vi "Configure Module.vi"(8 "error in (no error)":errorcluster, 10 "IOV ref in":refnum<k21>, 11 "Module Template in":refnum<class "SD Module.lvclass">) -> (0 "error out":errorcluster, 2 "IOV ref out":refnum<k21>, 3 "Module Template out":refnum<class "SD Module.lvclass">)   [LabVIEW 2017, in "Modules.lvlib" / "SD Module.lvclass"]
uses:
  SD Module.lvclass
  C:/Users/nitest/Documents/ni-official/niveristand-scan-engine-module-libraries/Source/RSI Module/RSI Module.lvclass
  SD Module.lvclass/SD Module.ctl
  <resource>/objmgr/cRIO.rc
  RSI Module/RSI Module.lvclass
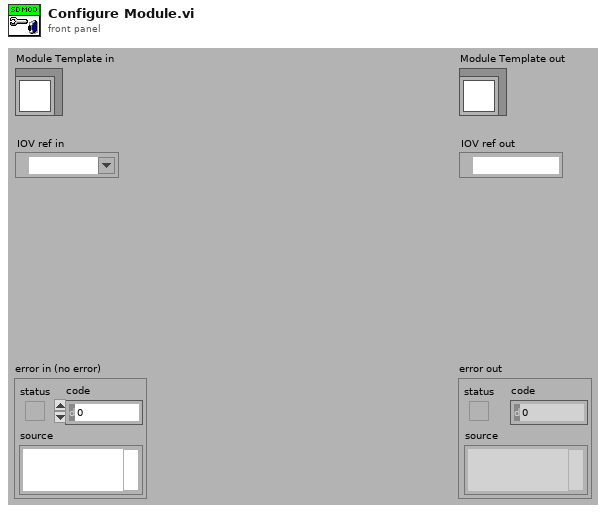
[diagram p1: front panel]
types:
  T1 = typedef "Modules.lvlib/SD Module.lvclass/Counter Channel.ctl" = cluster{"Measurement Mode":u32, "Count Edges":T2, "Period Measurement":T3, "Pulse Width Measurement":T4, "Frequency Measurement":T5}
  T2 = typedef "Modules.lvlib/SD Module.lvclass/Count Edges.ctl" = cluster{"Counter Event":u32, "Counter Source":u32, "Counter Direction":u32, "Terminal Count":u32, "Output Mode":u32, "Gate Mode":u32}
  T3 = typedef "Modules.lvlib/SD Module.lvclass/Period Measurement.ctl" = cluster{"Measurement Edge":u32}
  T4 = typedef "Modules.lvlib/SD Module.lvclass/Pulse Width Measurement.ctl" = cluster{"Measurement Type":u32}
  T5 = typedef "Modules.lvlib/SD Module.lvclass/Frequency Measurement.ctl" = cluster{"Measurement Edge":u32, "Measurement Timebase":u32}
  T6 = typedef "Modules.lvlib/SD Module.lvclass/CDO Channel.ctl" = cluster{"Counter driven enabled":bool}
  T7 = typedef "Modules.lvlib/SD Module.lvclass/PWM Channel.ctl" = cluster{"PWM frequency":u32}
  T8 = typedef "Modules.lvlib/SD Module.lvclass/Quadrature Channel.ctl" = cluster{"Timebase":u32, "Index Mode":u32}
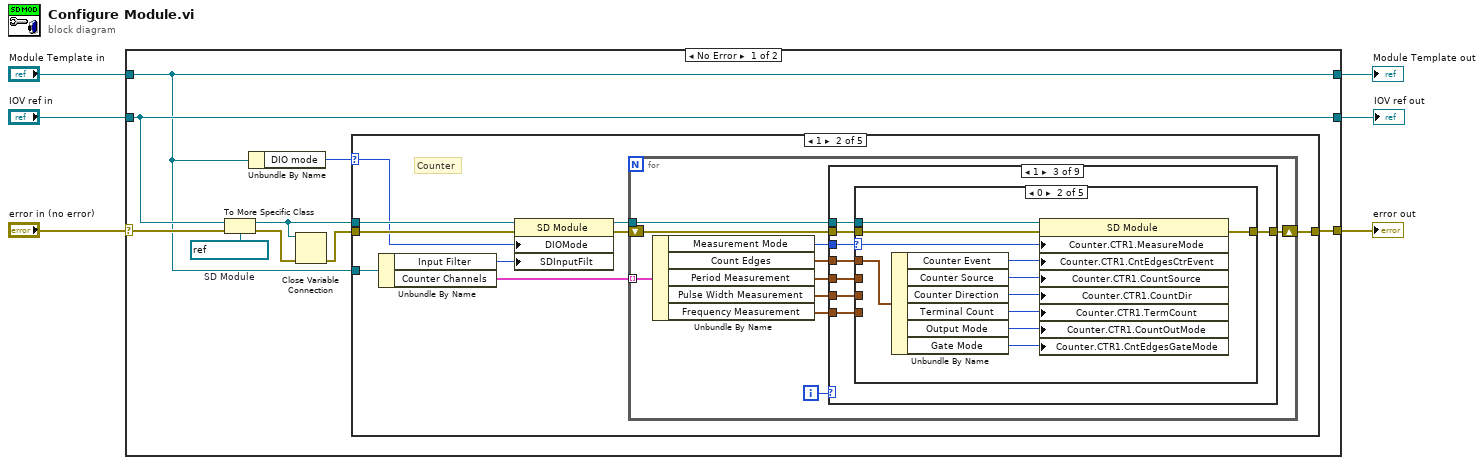
[diagram p0: block diagram]
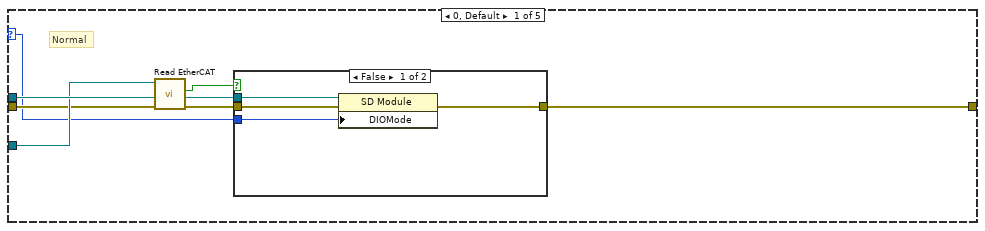
[diagram p2: hidden frame]
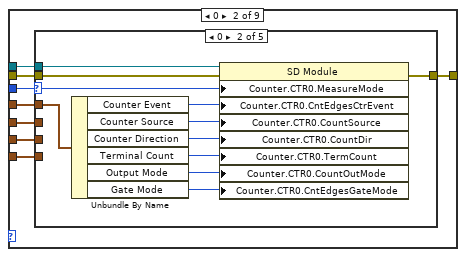
[diagram p5: hidden frame]
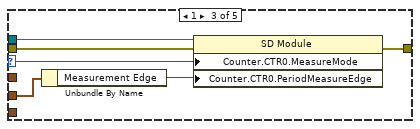
[diagram p7: hidden frame]
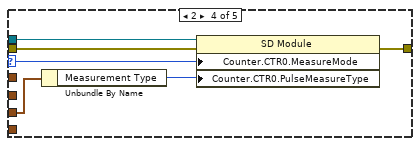
[diagram p8: hidden frame]
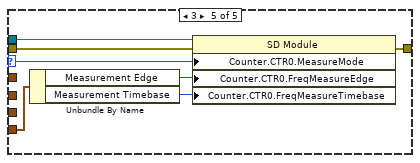
[diagram p9: hidden frame]
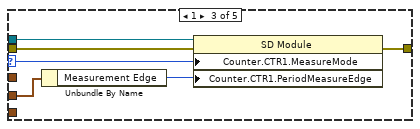
[diagram p11: hidden frame]
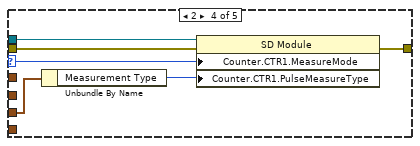
[diagram p12: hidden frame]
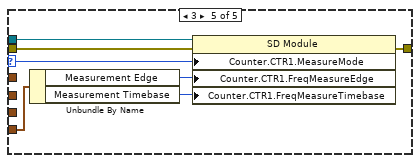
[diagram p13: hidden frame]
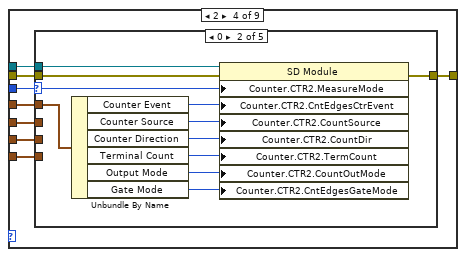
[diagram p14: hidden frame]
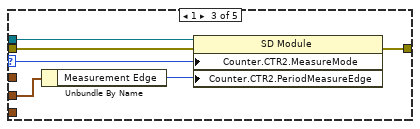
[diagram p16: hidden frame]
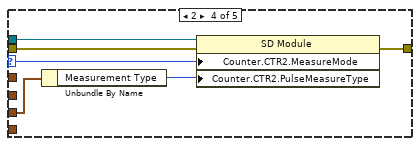
[diagram p17: hidden frame]
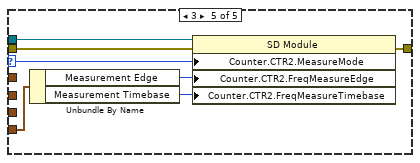
[diagram p18: hidden frame]
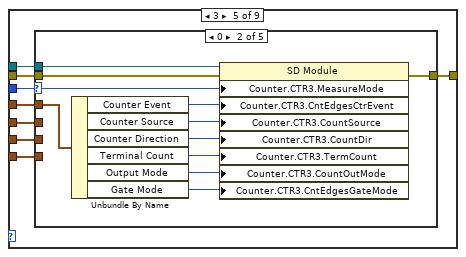
[diagram p19: hidden frame]
diagram:
  n1 = case shown="No Error" "error in (no error)" {
    selector: "error in (no error)" -> [w15 w484]
    tunnel: [w7 w484] -> w5
    tunnel: [w8 w483] -> w3
    tunnel: "Module Template in" -> [w8 w483]
    tunnel: "IOV ref in" -> [w13 w482]
    tunnel: [w13 w482] -> w1
    frame No Error {
      w14 = refnum<k21> refnum  # SD Module
      n2 = To More Specific Class(target class=w14, reference=w13, error in=w15) -> (specific class reference=w10:refnum<k21>, error out=w12:errorcluster)
      n3 = Unbundle By Name(w8) -> ("DIO mode"=w11:u32)
      n4 = Close Variable Connection(8:w12, 11:w10) -> (0:w9:errorcluster)
      n5 = case shown="1" w11 {
        selector: w11 -> [w16 w34 w366 w413 w461]
        tunnel: w10 -> [w22 w36 w368 w415 w463]
        tunnel: w9 -> [w18 w35 w367 w414 w462]
        tunnel: w8 -> [w20 w33 w365 w412 w460]
        tunnel: [w21 w28 w360 w408 w455] -> w7
        frame 0, Default {
          # "Normal"
          n6 = call "Read EtherCAT.vi"("error in (no error)"=w18, "RSI Module in"=w20) -> ("error out"=w17:errorcluster, "EtherCAT?"=w19:bool)  [unwired: 7 in, 1 out]
          n7 = case shown="False" w19 {
            tunnel: w22 -> [w26 _]
            tunnel: w17 -> [w25 w27]
            tunnel: [w24 w27] -> w21
            tunnel: w16 -> [w23 _]
            frame False {
              n8 = property class="SD Module"(reference=w26, error in=w25, "DIOMode"=w23) -> (error out=w24:errorcluster)  [unwired: 1 out]
            }
            frame True {
              # "Specialty Digital is not supported over\nEtherCAT, and explicitly configuring modules\nto use normal DIO mode will fail as a result."
            }
          }
        }
        frame 1 {
          # "Counter"
          n9 = Unbundle By Name(w33) -> ("Input Filter"=w32:u32, "Counter Channels"=w31:T1[])
          n10 = property class="SD Module"(reference=w36, error in=w35, "DIOMode"=w34, "SDInputFilt"=w32) -> (reference out=w30:refnum<k21>, error out=w29:errorcluster)
          n11 = for {
            tunnel: w31 -> [w42] mode=indexing
            tunnel: w30 -> [w45]
            shift-right: [w43] -> w28
            shift-left: w29 -> [w44]
            i -> [w46]
            n12 = Unbundle By Name(w42) -> ("Measurement Mode"=w41:u32, "Count Edges"=w40:T2, "Period Measurement"=w39:T3, "Pulse Width Measurement"=w38:T4, "Frequency Measurement"=w37:T5)
            n13 = case shown="1" w46 {
              tunnel: w45 -> [_ w50 w89 w128 w167 w206 w245 w284 w323]
              tunnel: w44 -> [w47 w49 w88 w127 w166 w205 w244 w283 w322]
              tunnel: [w47 w48 w87 w126 w165 w204 w243 w282 w321] -> w43
              tunnel: w41 -> [_ w55 w94 w133 w172 w211 w250 w289 w328]
              tunnel: w40 -> [_ w54 w93 w132 w171 w210 w249 w288 w327]
              tunnel: w39 -> [_ w53 w92 w131 w170 w209 w248 w287 w326]
              tunnel: w38 -> [_ w52 w91 w130 w169 w208 w247 w286 w325]
              tunnel: w37 -> [_ w51 w90 w129 w168 w207 w246 w285 w324]
              frame Default {
              }
              frame 0 {
                n14 = case shown="0" w55 {
                  selector: w55 -> [_ w64 w71 w77 w84]
                  tunnel: w54 -> [_ w67 _ _ _]
                  tunnel: w53 -> [_ _ w68 _ _]
                  tunnel: w52 -> [_ _ _ w74 _]
                  tunnel: w51 -> [_ _ _ _ w81]
                  tunnel: w50 -> [_ w66 w73 w79 w86]
                  tunnel: w49 -> [w56 w65 w72 w78 w85]
                  tunnel: [w56 w57 w69 w75 w82] -> w48
                  frame Default {
                  }
                  frame 0 {
                    n15 = Unbundle By Name(w67) -> ("Counter Event"=w63:u32, "Counter Source"=w62:u32, "Counter Direction"=w61:u32, "Terminal Count"=w60:u32, "Output Mode"=w59:u32, "Gate Mode"=w58:u32)
                    n16 = property class="SD Module"(reference=w66, error in=w65, "Counter.CTR0.MeasureMode"=w64, "Counter.CTR0.CntEdgesCtrEvent"=w63, "Counter.CTR0.CountSource"=w62, "Counter.CTR0.CountDir"=w61, "Counter.CTR0.TermCount"=w60, "Counter.CTR0.CountOutMode"=w59, "Counter.CTR0.CntEdgesGateMode"=w58) -> (error out=w57:errorcluster)  [unwired: 1 out]
                  }
                  frame 1 {
                    n17 = Unbundle By Name(w68) -> ("Measurement Edge"=w70:u32)
                    n18 = property class="SD Module"(reference=w73, error in=w72, "Counter.CTR0.MeasureMode"=w71, "Counter.CTR0.PeriodMeasureEdge"=w70) -> (error out=w69:errorcluster)  [unwired: 1 out]
                  }
                  frame 2 {
                    n19 = Unbundle By Name(w74) -> ("Measurement Type"=w76:u32)
                    n20 = property class="SD Module"(reference=w79, error in=w78, "Counter.CTR0.MeasureMode"=w77, "Counter.CTR0.PulseMeasureType"=w76) -> (error out=w75:errorcluster)  [unwired: 1 out]
                  }
                  frame 3 {
                    n21 = Unbundle By Name(w81) -> ("Measurement Edge"=w83:u32, "Measurement Timebase"=w80:u32)
                    n22 = property class="SD Module"(reference=w86, error in=w85, "Counter.CTR0.MeasureMode"=w84, "Counter.CTR0.FreqMeasureEdge"=w83, "Counter.CTR0.FreqMeasureTimebase"=w80) -> (error out=w82:errorcluster)  [unwired: 1 out]
                  }
                }
              }
              frame 1 {
                n23 = case shown="0" w94 {
                  selector: w94 -> [_ w103 w110 w116 w123]
                  tunnel: w93 -> [_ w106 _ _ _]
                  tunnel: w92 -> [_ _ w107 _ _]
                  tunnel: w91 -> [_ _ _ w113 _]
                  tunnel: w90 -> [_ _ _ _ w120]
                  tunnel: w89 -> [_ w105 w112 w118 w125]
                  tunnel: w88 -> [w95 w104 w111 w117 w124]
                  tunnel: [w95 w96 w108 w114 w121] -> w87
                  frame Default {
                  }
                  frame 0 {
                    n24 = Unbundle By Name(w106) -> ("Counter Event"=w102:u32, "Counter Source"=w101:u32, "Counter Direction"=w100:u32, "Terminal Count"=w99:u32, "Output Mode"=w98:u32, "Gate Mode"=w97:u32)
                    n25 = property class="SD Module"(reference=w105, error in=w104, "Counter.CTR1.MeasureMode"=w103, "Counter.CTR1.CntEdgesCtrEvent"=w102, "Counter.CTR1.CountSource"=w101, "Counter.CTR1.CountDir"=w100, "Counter.CTR1.TermCount"=w99, "Counter.CTR1.CountOutMode"=w98, "Counter.CTR1.CntEdgesGateMode"=w97) -> (error out=w96:errorcluster)  [unwired: 1 out]
                  }
                  frame 1 {
                    n26 = Unbundle By Name(w107) -> ("Measurement Edge"=w109:u32)
                    n27 = property class="SD Module"(reference=w112, error in=w111, "Counter.CTR1.MeasureMode"=w110, "Counter.CTR1.PeriodMeasureEdge"=w109) -> (error out=w108:errorcluster)  [unwired: 1 out]
                  }
                  frame 2 {
                    n28 = Unbundle By Name(w113) -> ("Measurement Type"=w115:u32)
                    n29 = property class="SD Module"(reference=w118, error in=w117, "Counter.CTR1.MeasureMode"=w116, "Counter.CTR1.PulseMeasureType"=w115) -> (error out=w114:errorcluster)  [unwired: 1 out]
                  }
                  frame 3 {
                    n30 = Unbundle By Name(w120) -> ("Measurement Edge"=w122:u32, "Measurement Timebase"=w119:u32)
                    n31 = property class="SD Module"(reference=w125, error in=w124, "Counter.CTR1.MeasureMode"=w123, "Counter.CTR1.FreqMeasureEdge"=w122, "Counter.CTR1.FreqMeasureTimebase"=w119) -> (error out=w121:errorcluster)  [unwired: 1 out]
                  }
                }
              }
              frame 2 {
                n32 = case shown="0" w133 {
                  selector: w133 -> [_ w142 w149 w155 w162]
                  tunnel: w132 -> [_ w145 _ _ _]
                  tunnel: w131 -> [_ _ w146 _ _]
                  tunnel: w130 -> [_ _ _ w152 _]
                  tunnel: w129 -> [_ _ _ _ w159]
                  tunnel: w128 -> [_ w144 w151 w157 w164]
                  tunnel: w127 -> [w134 w143 w150 w156 w163]
                  tunnel: [w134 w135 w147 w153 w160] -> w126
                  frame Default {
                  }
                  frame 0 {
                    n33 = Unbundle By Name(w145) -> ("Counter Event"=w141:u32, "Counter Source"=w140:u32, "Counter Direction"=w139:u32, "Terminal Count"=w138:u32, "Output Mode"=w137:u32, "Gate Mode"=w136:u32)
                    n34 = property class="SD Module"(reference=w144, error in=w143, "Counter.CTR2.MeasureMode"=w142, "Counter.CTR2.CntEdgesCtrEvent"=w141, "Counter.CTR2.CountSource"=w140, "Counter.CTR2.CountDir"=w139, "Counter.CTR2.TermCount"=w138, "Counter.CTR2.CountOutMode"=w137, "Counter.CTR2.CntEdgesGateMode"=w136) -> (error out=w135:errorcluster)  [unwired: 1 out]
                  }
                  frame 1 {
                    n35 = Unbundle By Name(w146) -> ("Measurement Edge"=w148:u32)
                    n36 = property class="SD Module"(reference=w151, error in=w150, "Counter.CTR2.MeasureMode"=w149, "Counter.CTR2.PeriodMeasureEdge"=w148) -> (error out=w147:errorcluster)  [unwired: 1 out]
                  }
                  frame 2 {
                    n37 = Unbundle By Name(w152) -> ("Measurement Type"=w154:u32)
                    n38 = property class="SD Module"(reference=w157, error in=w156, "Counter.CTR2.MeasureMode"=w155, "Counter.CTR2.PulseMeasureType"=w154) -> (error out=w153:errorcluster)  [unwired: 1 out]
                  }
                  frame 3 {
                    n39 = Unbundle By Name(w159) -> ("Measurement Edge"=w161:u32, "Measurement Timebase"=w158:u32)
                    n40 = property class="SD Module"(reference=w164, error in=w163, "Counter.CTR2.MeasureMode"=w162, "Counter.CTR2.FreqMeasureEdge"=w161, "Counter.CTR2.FreqMeasureTimebase"=w158) -> (error out=w160:errorcluster)  [unwired: 1 out]
                  }
                }
              }
              frame 3 {
                n41 = case shown="0" w172 {
                  selector: w172 -> [_ w181 w188 w194 w201]
                  tunnel: w171 -> [_ w184 _ _ _]
                  tunnel: w170 -> [_ _ w185 _ _]
                  tunnel: w169 -> [_ _ _ w191 _]
                  tunnel: w168 -> [_ _ _ _ w198]
                  tunnel: w167 -> [_ w183 w190 w196 w203]
                  tunnel: w166 -> [w173 w182 w189 w195 w202]
                  tunnel: [w173 w174 w186 w192 w199] -> w165
                  frame Default {
                  }
                  frame 0 {
                    n42 = Unbundle By Name(w184) -> ("Counter Event"=w180:u32, "Counter Source"=w179:u32, "Counter Direction"=w178:u32, "Terminal Count"=w177:u32, "Output Mode"=w176:u32, "Gate Mode"=w175:u32)
                    n43 = property class="SD Module"(reference=w183, error in=w182, "Counter.CTR3.MeasureMode"=w181, "Counter.CTR3.CntEdgesCtrEvent"=w180, "Counter.CTR3.CountSource"=w179, "Counter.CTR3.CountDir"=w178, "Counter.CTR3.TermCount"=w177, "Counter.CTR3.CountOutMode"=w176, "Counter.CTR3.CntEdgesGateMode"=w175) -> (error out=w174:errorcluster)  [unwired: 1 out]
                  }
                  frame 1 {
                    n44 = Unbundle By Name(w185) -> ("Measurement Edge"=w187:u32)
                    n45 = property class="SD Module"(reference=w190, error in=w189, "Counter.CTR3.MeasureMode"=w188, "Counter.CTR3.PeriodMeasureEdge"=w187) -> (error out=w186:errorcluster)  [unwired: 1 out]
                  }
                  frame 2 {
                    n46 = Unbundle By Name(w191) -> ("Measurement Type"=w193:u32)
                    n47 = property class="SD Module"(reference=w196, error in=w195, "Counter.CTR3.MeasureMode"=w194, "Counter.CTR3.PulseMeasureType"=w193) -> (error out=w192:errorcluster)  [unwired: 1 out]
                  }
                  frame 3 {
                    n48 = Unbundle By Name(w198) -> ("Measurement Edge"=w200:u32, "Measurement Timebase"=w197:u32)
                    n49 = property class="SD Module"(reference=w203, error in=w202, "Counter.CTR3.MeasureMode"=w201, "Counter.CTR3.FreqMeasureEdge"=w200, "Counter.CTR3.FreqMeasureTimebase"=w197) -> (error out=w199:errorcluster)  [unwired: 1 out]
                  }
                }
              }
              frame 4 {
                n50 = case shown="0" w211 {
                  selector: w211 -> [_ w220 w227 w233 w240]
                  tunnel: w210 -> [_ w223 _ _ _]
                  tunnel: w209 -> [_ _ w224 _ _]
                  tunnel: w208 -> [_ _ _ w230 _]
                  tunnel: w207 -> [_ _ _ _ w237]
                  tunnel: w206 -> [_ w222 w229 w235 w242]
                  tunnel: w205 -> [w212 w221 w228 w234 w241]
                  tunnel: [w212 w213 w225 w231 w238] -> w204
                  frame Default {
                  }
                  frame 0 {
                    n51 = Unbundle By Name(w223) -> ("Counter Event"=w219:u32, "Counter Source"=w218:u32, "Counter Direction"=w217:u32, "Terminal Count"=w216:u32, "Output Mode"=w215:u32, "Gate Mode"=w214:u32)
                    n52 = property class="SD Module"(reference=w222, error in=w221, "Counter.CTR4.MeasureMode"=w220, "Counter.CTR4.CntEdgesCtrEvent"=w219, "Counter.CTR4.CountSource"=w218, "Counter.CTR4.CountDir"=w217, "Counter.CTR4.TermCount"=w216, "Counter.CTR4.CountOutMode"=w215, "Counter.CTR4.CntEdgesGateMode"=w214) -> (error out=w213:errorcluster)  [unwired: 1 out]
                  }
                  frame 1 {
                    n53 = Unbundle By Name(w224) -> ("Measurement Edge"=w226:u32)
                    n54 = property class="SD Module"(reference=w229, error in=w228, "Counter.CTR4.MeasureMode"=w227, "Counter.CTR4.PeriodMeasureEdge"=w226) -> (error out=w225:errorcluster)  [unwired: 1 out]
                  }
                  frame 2 {
                    n55 = Unbundle By Name(w230) -> ("Measurement Type"=w232:u32)
                    n56 = property class="SD Module"(reference=w235, error in=w234, "Counter.CTR4.MeasureMode"=w233, "Counter.CTR4.PulseMeasureType"=w232) -> (error out=w231:errorcluster)  [unwired: 1 out]
                  }
                  frame 3 {
                    n57 = Unbundle By Name(w237) -> ("Measurement Edge"=w239:u32, "Measurement Timebase"=w236:u32)
                    n58 = property class="SD Module"(reference=w242, error in=w241, "Counter.CTR4.MeasureMode"=w240, "Counter.CTR4.FreqMeasureEdge"=w239, "Counter.CTR4.FreqMeasureTimebase"=w236) -> (error out=w238:errorcluster)  [unwired: 1 out]
                  }
                }
              }
              frame 5 {
                n59 = case shown="0" w250 {
                  selector: w250 -> [_ w259 w266 w272 w279]
                  tunnel: w249 -> [_ w262 _ _ _]
                  tunnel: w248 -> [_ _ w263 _ _]
                  tunnel: w247 -> [_ _ _ w269 _]
                  tunnel: w246 -> [_ _ _ _ w276]
                  tunnel: w245 -> [_ w261 w268 w274 w281]
                  tunnel: w244 -> [w251 w260 w267 w273 w280]
                  tunnel: [w251 w252 w264 w270 w277] -> w243
                  frame Default {
                  }
                  frame 0 {
                    n60 = Unbundle By Name(w262) -> ("Counter Event"=w258:u32, "Counter Source"=w257:u32, "Counter Direction"=w256:u32, "Terminal Count"=w255:u32, "Output Mode"=w254:u32, "Gate Mode"=w253:u32)
                    n61 = property class="SD Module"(reference=w261, error in=w260, "Counter.CTR5.MeasureMode"=w259, "Counter.CTR5.CntEdgesCtrEvent"=w258, "Counter.CTR5.CountSource"=w257, "Counter.CTR5.CountDir"=w256, "Counter.CTR5.TermCount"=w255, "Counter.CTR5.CountOutMode"=w254, "Counter.CTR5.CntEdgesGateMode"=w253) -> (error out=w252:errorcluster)  [unwired: 1 out]
                  }
                  frame 1 {
                    n62 = Unbundle By Name(w263) -> ("Measurement Edge"=w265:u32)
                    n63 = property class="SD Module"(reference=w268, error in=w267, "Counter.CTR5.MeasureMode"=w266, "Counter.CTR5.PeriodMeasureEdge"=w265) -> (error out=w264:errorcluster)  [unwired: 1 out]
                  }
                  frame 2 {
                    n64 = Unbundle By Name(w269) -> ("Measurement Type"=w271:u32)
                    n65 = property class="SD Module"(reference=w274, error in=w273, "Counter.CTR5.MeasureMode"=w272, "Counter.CTR5.PulseMeasureType"=w271) -> (error out=w270:errorcluster)  [unwired: 1 out]
                  }
                  frame 3 {
                    n66 = Unbundle By Name(w276) -> ("Measurement Edge"=w278:u32, "Measurement Timebase"=w275:u32)
                    n67 = property class="SD Module"(reference=w281, error in=w280, "Counter.CTR5.MeasureMode"=w279, "Counter.CTR5.FreqMeasureEdge"=w278, "Counter.CTR5.FreqMeasureTimebase"=w275) -> (error out=w277:errorcluster)  [unwired: 1 out]
                  }
                }
              }
              frame 6 {
                n68 = case shown="0" w289 {
                  selector: w289 -> [_ w298 w305 w311 w318]
                  tunnel: w288 -> [_ w301 _ _ _]
                  tunnel: w287 -> [_ _ w302 _ _]
                  tunnel: w286 -> [_ _ _ w308 _]
                  tunnel: w285 -> [_ _ _ _ w315]
                  tunnel: w284 -> [_ w300 w307 w313 w320]
                  tunnel: w283 -> [w290 w299 w306 w312 w319]
                  tunnel: [w290 w291 w303 w309 w316] -> w282
                  frame Default {
                  }
                  frame 0 {
                    n69 = Unbundle By Name(w301) -> ("Counter Event"=w297:u32, "Counter Source"=w296:u32, "Counter Direction"=w295:u32, "Terminal Count"=w294:u32, "Output Mode"=w293:u32, "Gate Mode"=w292:u32)
                    n70 = property class="SD Module"(reference=w300, error in=w299, "Counter.CTR6.MeasureMode"=w298, "Counter.CTR6.CntEdgesCtrEvent"=w297, "Counter.CTR6.CountSource"=w296, "Counter.CTR6.CountDir"=w295, "Counter.CTR6.TermCount"=w294, "Counter.CTR6.CountOutMode"=w293, "Counter.CTR6.CntEdgesGateMode"=w292) -> (error out=w291:errorcluster)  [unwired: 1 out]
                  }
                  frame 1 {
                    n71 = Unbundle By Name(w302) -> ("Measurement Edge"=w304:u32)
                    n72 = property class="SD Module"(reference=w307, error in=w306, "Counter.CTR6.MeasureMode"=w305, "Counter.CTR6.PeriodMeasureEdge"=w304) -> (error out=w303:errorcluster)  [unwired: 1 out]
                  }
                  frame 2 {
                    n73 = Unbundle By Name(w308) -> ("Measurement Type"=w310:u32)
                    n74 = property class="SD Module"(reference=w313, error in=w312, "Counter.CTR6.MeasureMode"=w311, "Counter.CTR6.PulseMeasureType"=w310) -> (error out=w309:errorcluster)  [unwired: 1 out]
                  }
                  frame 3 {
                    n75 = Unbundle By Name(w315) -> ("Measurement Edge"=w317:u32, "Measurement Timebase"=w314:u32)
                    n76 = property class="SD Module"(reference=w320, error in=w319, "Counter.CTR6.MeasureMode"=w318, "Counter.CTR6.FreqMeasureEdge"=w317, "Counter.CTR6.FreqMeasureTimebase"=w314) -> (error out=w316:errorcluster)  [unwired: 1 out]
                  }
                }
              }
              frame 7 {
                n77 = case shown="0" w328 {
                  selector: w328 -> [_ w337 w344 w350 w357]
                  tunnel: w327 -> [_ w340 _ _ _]
                  tunnel: w326 -> [_ _ w341 _ _]
                  tunnel: w325 -> [_ _ _ w347 _]
                  tunnel: w324 -> [_ _ _ _ w354]
                  tunnel: w323 -> [_ w339 w346 w352 w359]
                  tunnel: w322 -> [w329 w338 w345 w351 w358]
                  tunnel: [w329 w330 w342 w348 w355] -> w321
                  frame Default {
                  }
                  frame 0 {
                    n78 = Unbundle By Name(w340) -> ("Counter Event"=w336:u32, "Counter Source"=w335:u32, "Counter Direction"=w334:u32, "Terminal Count"=w333:u32, "Output Mode"=w332:u32, "Gate Mode"=w331:u32)
                    n79 = property class="SD Module"(reference=w339, error in=w338, "Counter.CTR7.MeasureMode"=w337, "Counter.CTR7.CntEdgesCtrEvent"=w336, "Counter.CTR7.CountSource"=w335, "Counter.CTR7.CountDir"=w334, "Counter.CTR7.TermCount"=w333, "Counter.CTR7.CountOutMode"=w332, "Counter.CTR7.CntEdgesGateMode"=w331) -> (error out=w330:errorcluster)  [unwired: 1 out]
                  }
                  frame 1 {
                    n80 = Unbundle By Name(w341) -> ("Measurement Edge"=w343:u32)
                    n81 = property class="SD Module"(reference=w346, error in=w345, "Counter.CTR7.MeasureMode"=w344, "Counter.CTR7.PeriodMeasureEdge"=w343) -> (error out=w342:errorcluster)  [unwired: 1 out]
                  }
                  frame 2 {
                    n82 = Unbundle By Name(w347) -> ("Measurement Type"=w349:u32)
                    n83 = property class="SD Module"(reference=w352, error in=w351, "Counter.CTR7.MeasureMode"=w350, "Counter.CTR7.PulseMeasureType"=w349) -> (error out=w348:errorcluster)  [unwired: 1 out]
                  }
                  frame 3 {
                    n84 = Unbundle By Name(w354) -> ("Measurement Edge"=w356:u32, "Measurement Timebase"=w353:u32)
                    n85 = property class="SD Module"(reference=w359, error in=w358, "Counter.CTR7.MeasureMode"=w357, "Counter.CTR7.FreqMeasureEdge"=w356, "Counter.CTR7.FreqMeasureTimebase"=w353) -> (error out=w355:errorcluster)  [unwired: 1 out]
                  }
                }
              }
            }
          }
        }
        frame 2 {
          # "Counter-Driven Output"
          n86 = Unbundle By Name(w365) -> ("Drive From Slot"=w362:u32, "CDO Channels"=w361:T6[])
          n87 = property class="SD Module"(reference=w368, error in=w367, "DIOMode"=w366, "CDO.CountSlvMastSlot"=w362) -> (reference out=w364:refnum<k21>, error out=w363:errorcluster)
          n88 = for {
            tunnel: w364 -> [w373]
            shift-right: [w371] -> w360
            shift-left: w363 -> [w372]
            tunnel: w361 -> [w369] mode=indexing
            i -> [w374]
            n89 = Unbundle By Name(w369) -> ("Counter driven enabled"=w370:bool)
            n90 = case shown="0" w374 {
              tunnel: w373 -> [_ w379 w383 w387 w391 w395 w399 w403 w407]
              tunnel: w372 -> [w375 w378 w382 w386 w390 w394 w398 w402 w406]
              tunnel: [w375 w377 w381 w385 w389 w393 w397 w401 w405] -> w371
              tunnel: w370 -> [_ w376 w380 w384 w388 w392 w396 w400 w404]
              frame Default {
              }
              frame 0 {
                n91 = property class="SD Module"(reference=w379, error in=w378, "CDO.CTR0.CtrDrivenEnabled"=w376) -> (error out=w377:errorcluster)  [unwired: 1 out]
              }
              frame 1 {
                n92 = property class="SD Module"(reference=w383, error in=w382, "CDO.CTR1.CtrDrivenEnabled"=w380) -> (error out=w381:errorcluster)  [unwired: 1 out]
              }
              frame 2 {
                n93 = property class="SD Module"(reference=w387, error in=w386, "CDO.CTR2.CtrDrivenEnabled"=w384) -> (error out=w385:errorcluster)  [unwired: 1 out]
              }
              frame 3 {
                n94 = property class="SD Module"(reference=w391, error in=w390, "CDO.CTR3.CtrDrivenEnabled"=w388) -> (error out=w389:errorcluster)  [unwired: 1 out]
              }
              frame 4 {
                n95 = property class="SD Module"(reference=w395, error in=w394, "CDO.CTR4.CtrDrivenEnabled"=w392) -> (error out=w393:errorcluster)  [unwired: 1 out]
              }
              frame 5 {
                n96 = property class="SD Module"(reference=w399, error in=w398, "CDO.CTR5.CtrDrivenEnabled"=w396) -> (error out=w397:errorcluster)  [unwired: 1 out]
              }
              frame 6 {
                n97 = property class="SD Module"(reference=w403, error in=w402, "CDO.CTR6.CtrDrivenEnabled"=w400) -> (error out=w401:errorcluster)  [unwired: 1 out]
              }
              frame 7 {
                n98 = property class="SD Module"(reference=w407, error in=w406, "CDO.CTR7.CtrDrivenEnabled"=w404) -> (error out=w405:errorcluster)  [unwired: 1 out]
              }
            }
          }
        }
        frame 3 {
          # "Pulse-Width Modulation"
          n99 = Unbundle By Name(w412) -> ("PWM Channels"=w409:T7[])
          n100 = property class="SD Module"(reference=w415, error in=w414, "DIOMode"=w413) -> (reference out=w411:refnum<k21>, error out=w410:errorcluster)
          n101 = for {
            tunnel: w411 -> [w420]
            shift-right: [w418] -> w408
            shift-left: w410 -> [w419]
            tunnel: w409 -> [w416] mode=indexing
            i -> [w421]
            n102 = Unbundle By Name(w416) -> ("PWM frequency"=w417:u32)
            n103 = case shown="0" w421 {
              tunnel: w420 -> [_ w426 w430 w434 w438 w442 w446 w450 w454]
              tunnel: w419 -> [w422 w425 w429 w433 w437 w441 w445 w449 w453]
              tunnel: [w422 w424 w428 w432 w436 w440 w444 w448 w452] -> w418
              tunnel: w417 -> [_ w423 w427 w431 w435 w439 w443 w447 w451]
              frame Default {
              }
              frame 0 {
                n104 = property class="SD Module"(reference=w426, error in=w425, "PWM.PWM0.PWMFrequency"=w423) -> (error out=w424:errorcluster)  [unwired: 1 out]
              }
              frame 1 {
                n105 = property class="SD Module"(reference=w430, error in=w429, "PWM.PWM1.PWMFrequency"=w427) -> (error out=w428:errorcluster)  [unwired: 1 out]
              }
              frame 2 {
                n106 = property class="SD Module"(reference=w434, error in=w433, "PWM.PWM2.PWMFrequency"=w431) -> (error out=w432:errorcluster)  [unwired: 1 out]
              }
              frame 3 {
                n107 = property class="SD Module"(reference=w438, error in=w437, "PWM.PWM3.PWMFrequency"=w435) -> (error out=w436:errorcluster)  [unwired: 1 out]
              }
              frame 4 {
                n108 = property class="SD Module"(reference=w442, error in=w441, "PWM.PWM4.PWMFrequency"=w439) -> (error out=w440:errorcluster)  [unwired: 1 out]
              }
              frame 5 {
                n109 = property class="SD Module"(reference=w446, error in=w445, "PWM.PWM5.PWMFrequency"=w443) -> (error out=w444:errorcluster)  [unwired: 1 out]
              }
              frame 6 {
                n110 = property class="SD Module"(reference=w450, error in=w449, "PWM.PWM6.PWMFrequency"=w447) -> (error out=w448:errorcluster)  [unwired: 1 out]
              }
              frame 7 {
                n111 = property class="SD Module"(reference=w454, error in=w453, "PWM.PWM7.PWMFrequency"=w451) -> (error out=w452:errorcluster)  [unwired: 1 out]
              }
            }
          }
        }
        frame 4 {
          # "Quadrature"
          n112 = Unbundle By Name(w460) -> ("Input Filter"=w459:u32, "Quadrature Channels"=w458:T8[])
          n113 = property class="SD Module"(reference=w463, error in=w462, "DIOMode"=w461, "SDInputFilt"=w459) -> (reference out=w457:refnum<k21>, error out=w456:errorcluster)
          n114 = for {
            tunnel: w458 -> [w466] mode=indexing
            tunnel: w457 -> [w469]
            shift-right: [w467] -> w455
            shift-left: w456 -> [w468]
            i -> [w470]
            n115 = Unbundle By Name(w466) -> ("Timebase"=w465:u32, "Index Mode"=w464:u32)
            n116 = case shown="0" w470 {
              tunnel: w469 -> [_ w476 w481]
              tunnel: w468 -> [w471 w475 w480]
              tunnel: [w471 w474 w479] -> w467
              tunnel: w465 -> [_ w473 w478]
              tunnel: w464 -> [_ w472 w477]
              frame Default {
              }
              frame 0 {
                n117 = property class="SD Module"(reference=w476, error in=w475, "Quad.Quadrature0.QuadTimebase"=w473, "Quad.Quadrature0.QuadIdxMode"=w472) -> (error out=w474:errorcluster)  [unwired: 1 out]
              }
              frame 1 {
                n118 = property class="SD Module"(reference=w481, error in=w480, "Quad.Quadrature1.QuadTimebase"=w478, "Quad.Quadrature0.QuadIdxMode"=w477) -> (error out=w479:errorcluster)  [unwired: 1 out]
              }
            }
          }
        }
      }
    }
    frame Error {
    }
  }
  "error out" <- w5
  "Module Template out" <- w3
  "IOV ref out" <- w1
